vi "Cluster Id Constant.vi"() -> (0 "cluster id env":string="NIDISCOVERY_CLUSTERID")   [LabVIEW 2021, in "NI Discovery V1 Client.lvlib"]
uses:
  NI Discovery V1 Client.lvlib
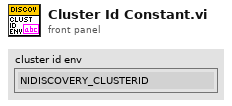
[diagram p1: front panel]
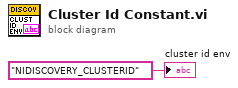
[diagram p0: block diagram]
diagram:
  "cluster id env" <- "NIDISCOVERY_CLUSTERID" ("name")
